vi "_Read.vi"(8 "errorIN":errorcluster caption="Error", 11 "LCD in":refnum<class "LCD Retarder.lvclass">) -> (0 "errorOUT":errorcluster caption="Error out", 2 "X array":T1, 3 "LCD out":refnum<class "LCD Retarder.lvclass">)   [LabVIEW 2009, in "LCD Retarder.lvclass"]
uses:
  LCD Retarder.lvclass
  Utility Classes/Readable/X array.ctl
  Utility Classes/Readable/X.ctl
  LCD Retarder.lvclass/LCD Retarder.ctl
  Utility Classes/Readable/Readable.lvclass
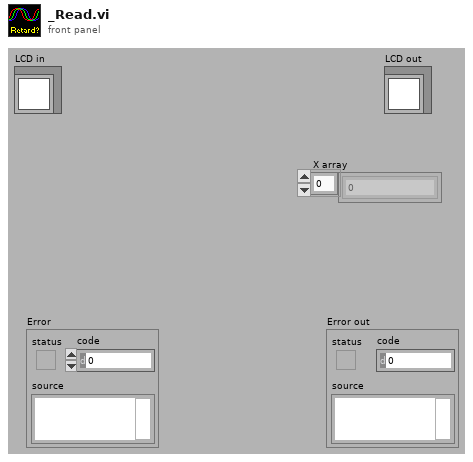
[diagram p1: front panel]
types:
  T1 = typedef "Readable.lvclass/X array.ctl" = T2[]
  T2 = typedef "Readable.lvclass/X.ctl" = dbl
  T3 = cluster{"Device Handle":u32, "Pipe 0 Handle":u32, "Pipe 1 Handle":u32}
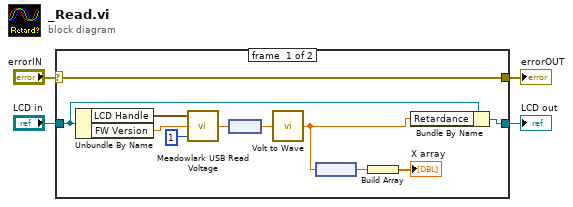
[diagram p0: block diagram]
diagram:
  n1 = case shown="No Error" "errorIN" {
    selector: "errorIN" -> [w9 w16]
    tunnel: [w15 w17] -> w4
    tunnel: "LCD in" -> [w14 w17]
    tunnel: [w9 w16] -> w1
    frame #0 {
      n2 = Unbundle By Name(w14) -> ("LCD Handle"=w12:T3, "FW Version"=w11:dbl)
      n3 = call "Meadowlark USB Read Voltage.VI"("LC Channel"=1, "FW Version"=w11, "USB Open Device Cluster"=w12) -> ("Readout \nVoltage"=w10:dbl)
      n4 = node(w10) -> (w7:dbl[unit])
      n5 = call "Volt to Wave.vi"("Voltage"=w7) -> ("Retardance"=w5:dbl[unit])
      n6 = node(w5) -> (w6:dbl)
      n7 = Build Array(w6) -> (→"X array":dbl[])
      n8 = Bundle By Name(cluster=w14, "Retardance"=w5) -> (w15:refnum<class "LCD Retarder.lvclass">)
    }
    frame #1 {
    }
  }
  "errorOUT" <- w1
  "LCD out" <- w4
